vi "Duplicate y Scale.vi"(8 "error in (no error)":errorcluster, 10 "Plot.Y Scale Index":u32[](array[numeric]), 11 "ACC,TC,SG 2":refnum<vi>) -> (0 "error out":errorcluster)   [LabVIEW 2022 SP3]
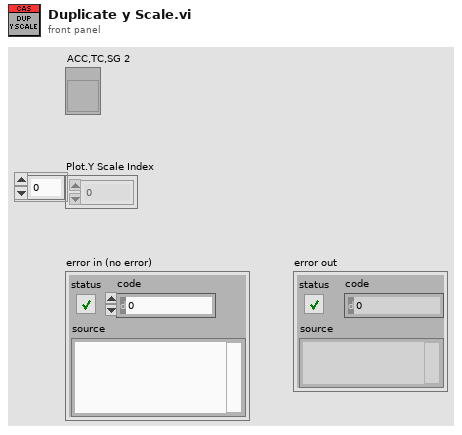
[diagram p1: front panel]
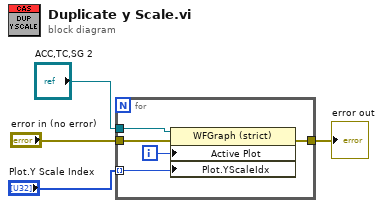
[diagram p0: block diagram]
diagram:
  n1 = for {
    tunnel: "error in (no error)" -> [w8]
    tunnel: [w9] -> w4
    tunnel: "ACC,TC,SG 2" -> [w7]
    tunnel: "Plot.Y Scale Index" -> [w6] mode=indexing
    i -> [w5]
    n2 = property class="WFGraph (strict)"(reference=w7, error in=w8, "Active Plot"=w5, "Plot.YScaleIdx"=w6) -> (error out=w9:errorcluster)  [unwired: 1 out]
  }
  "error out" <- w4
